vi "Actor Core.vi"(8 "error in":errorcluster, 11 "Supervisor in":refnum<class "Supervisor.lvclass">) -> (0 "error out":errorcluster, 3 "Actor out":refnum<class "Actor.lvclass">)   [LabVIEW 2020, in "Supervisor.lvlib" / "Supervisor.lvclass"]
doc: "<p>(<strong>Filename</strong>: <span class=\"dnl\">Actor Framework.lvlib:Actor.lvclass:Actor Core.vi</span>)</p>\n<p>Receives messages to the actor, reacts to them, and initiates any error handling that may shut the actor down.</p>\n<p>Descendant classes may override this VI to append parallel tasks for the actor to complete while it handles messages. Overrides use the <a href=\"nihelplauncher://docs/csh?context=lvcore_glang_udclass\">Call Parent Class Method</a> node.</p>"
uses:
  Supervisor.lvclass
  C:/Program Files/National Instruments/LabVIEW 2026/vi.lib/ActorFramework/Actor/Actor.lvclass
  <vilib>/ActorFramework/Actor/Actor.lvclass
  DAQ AI/DAQ AI/DAQ AI.lvclass
  DAQ DI/DAQ DI/DAQ DI.lvclass
  UI/UI/UI.lvclass
  <vilib>/ActorFramework/Message Enqueuer/Message Enqueuer.lvclass
  <vilib>/ActorFramework/Actor/Actor.lvclass/Actor.ctl
  <vilib>/ActorFramework/Message Enqueuer/Message Enqueuer.lvclass/Message Enqueuer.ctl
  Supervisor.lvclass/Supervisor.ctl
  DAQ AI/DAQ AI Messages/Threshold Msg/Threshold Msg.lvclass/Threshold Msg.ctl
  UI/UI Messages/Waveform Msg/Waveform Msg.lvclass/Waveform Msg.ctl
  UI/UI Messages/Status Msg/Status Msg.lvclass/Status Msg.ctl
  DAQ AI/DAQ AI Messages/Threshold Msg/Threshold Msg.lvclass
  C:/Program Files/National Instruments/LabVIEW 2026/vi.lib/ActorFramework/Message/Message.lvclass
  UI/UI Messages/Waveform Msg/Waveform Msg.lvclass
  UI/UI Messages/Status Msg/Status Msg.lvclass
  UI/UI Messages/Over Threshold Msg/Over Threshold Msg.lvclass
  DAQ DI/DAQ DI Messages/Acquire Status Msg/Acquire Status Msg.lvclass
  C:/Users/taacr/OneDrive/HP/Local/Actor Framework/Supervisor/Supervisor/Supervisor.lvclass
  C:/Users/taacr/OneDrive/HP/Local/Actor Framework/UI/UI/UI.lvclass
  C:/Users/taacr/OneDrive/HP/Local/Actor Framework/DAQ AI/DAQ AI/DAQ AI.lvclass
  C:/Users/taacr/OneDrive/HP/Local/Actor Framework/DAQ DI/DAQ DI/DAQ DI.lvclass
  TypeDef/Actor Queues.ctl
panel:
  out "Waveform Graph":waveform(dbl)[](graph)
  out "Threshold":dbl
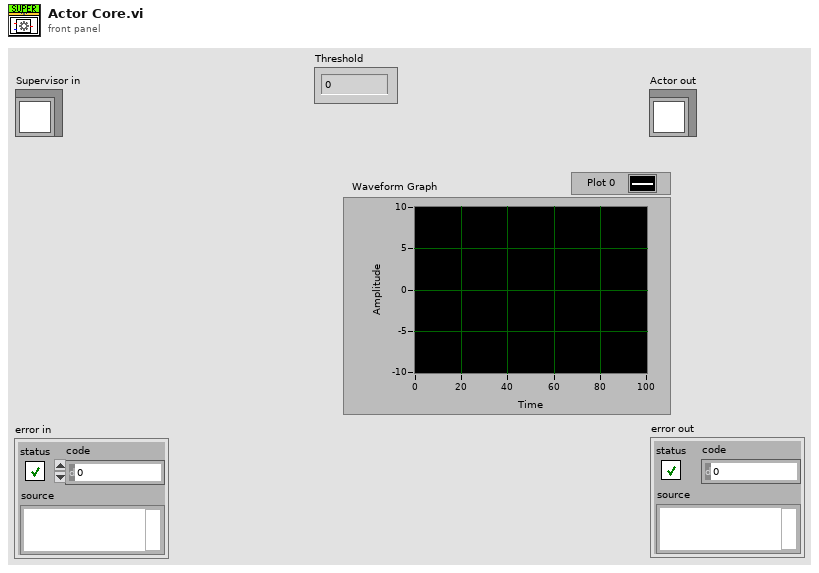
[diagram p1: front panel]
types:
  T1 = typedef "Supervisor.lvlib/Supervisor.lvclass/Actor Queues.ctl" = cluster{"Supervisor":refnum<class "Message Enqueuer.lvclass">, "UI":refnum<class "Message Enqueuer.lvclass">, "DAQ AI":refnum<class "Message Enqueuer.lvclass">, "DAQ DI":refnum<class "Message Enqueuer.lvclass">}
  T2 = typedef "Supervisor.lvlib/Supervisor.lvclass/User Events.ctl" = cluster{"Threshold Event":refnum<user-event>, "Waveform Graph Event":refnum<user-event>, "Status Event":refnum<user-event>, "Start/Stop Acquisition Event":refnum<user-event>, "Close UI Event":refnum<user-event>, "Stop Event":refnum<user-event>, "Over Threshold Event":refnum<user-event>}
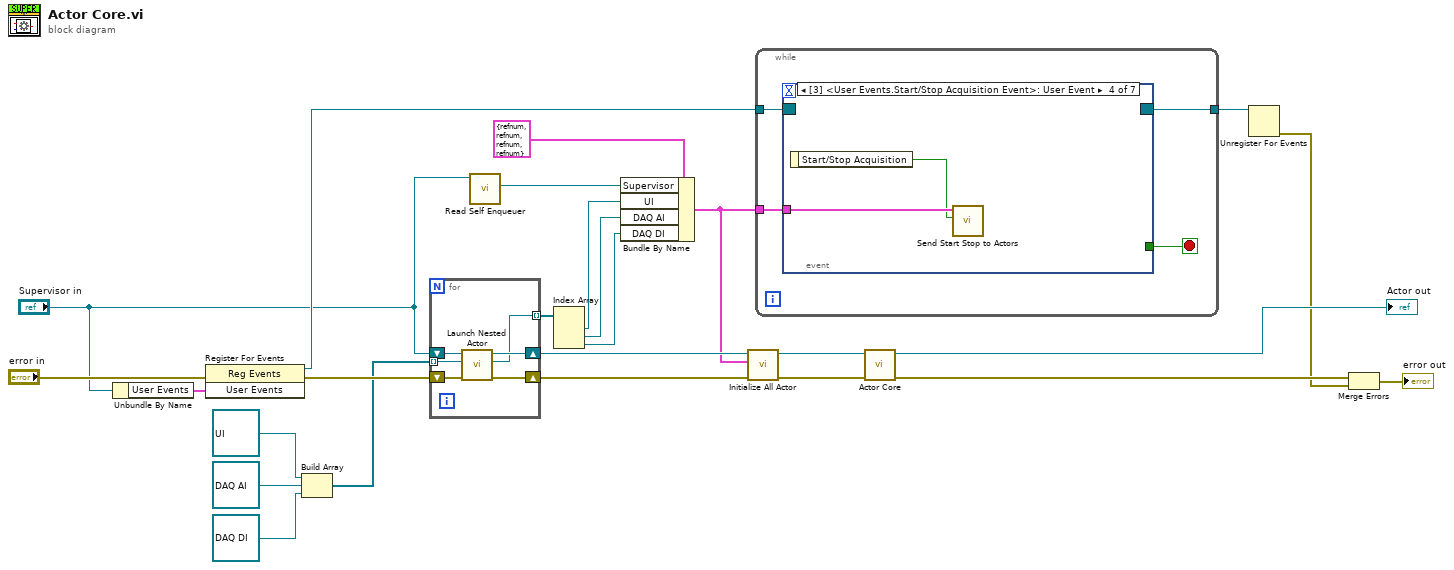
[diagram p0: block diagram]
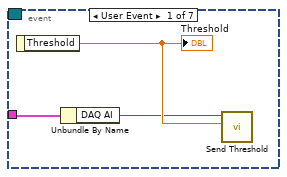
[diagram p2: hidden frame]
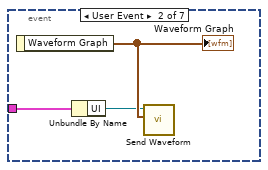
[diagram p3: hidden frame]
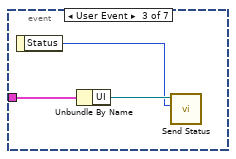
[diagram p4: hidden frame]
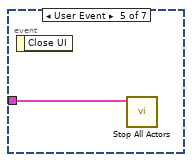
[diagram p5: hidden frame]
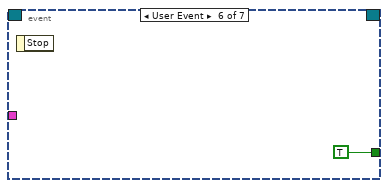
[diagram p6: hidden frame]
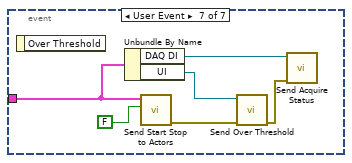
[diagram p7: hidden frame]
diagram:
  n1 = Unbundle By Name("Supervisor in") -> ("User Events"=w23:T2)
  n2 = register-events(error in="error in", w23) -> (reference out=w22:refnum<event-registration>, error out=w20:errorcluster)  [unwired: 1 in]
  n3 = Build Array(refnum<class "UI.lvclass"> refnum ("UI.lvlib:UI.lvclass"), refnum<class "DAQ AI.lvclass"> refnum ("DAQ AI.lvclass"), refnum<class "DAQ DI.lvclass"> refnum ("DAQ DI.lvlib:DAQ DI.lvclass")) -> (w19:refnum<class "Actor.lvclass">[])
  n4 = for {
    shift-right: [w29] -> w11
    shift-left: "Supervisor in" -> [w31]
    shift-right: [w28] -> w10
    shift-left: w20 -> [w30]
    tunnel: w19 -> [w27] mode=indexing
    tunnel: [w26] -> w15 mode=indexing
    n5 = call <vilib>:"Launch Nested Actor.vi"("error in (no error)"=w30, "Nested Actor"=w27, "Caller Actor in"=w31) -> ("error out"=w28:errorcluster, "Nested Actor's Enqueuer"=w26:refnum<class "Message Enqueuer.lvclass">, "Caller Actor out"=w29:refnum<class "Supervisor.lvclass">)  [unwired: 6 in]
  }
  n6 = call <vilib>:"Read Self Enqueuer.vi"("Actor"="Supervisor in") -> ("Self Enqueuer"=w16:refnum<class "Message Enqueuer.lvclass">)  [unwired: 10 in]
  n7 = Index Array(array=w15) -> (element #1=w14:refnum<class "Message Enqueuer.lvclass">, element #2=w13:refnum<class "Message Enqueuer.lvclass">, element #3=w12:refnum<class "Message Enqueuer.lvclass">)  [unwired: 3 in]
  n8 = Bundle By Name(cluster=T1 {"Supervisor"=refnum, "UI"=refnum, "DAQ AI"=refnum, "DAQ DI"=refnum} ("Actor Queue"), "Supervisor"=w16, "UI"=w14, "DAQ AI"=w13, "DAQ DI"=w12) -> (w7:T1)
  n9 = call "Initialize All Actor.vi"("error in (no error)"=w10, "Actor Queues"=w7, "Supervisor in"=w11) -> ("error out"=w8:errorcluster, "Supervisor out"=w9:refnum<class "Supervisor.lvclass">)  [unwired: 7 in]
  n10 = while {
    tunnel: w22 -> [w35]
    tunnel: w7 -> [w34]
    tunnel: [w33] -> w6
    stop <- w32 stop-if-true
    n11 = event shown="[3] <User Events.Start/Stop Acquisition Event>: User Event" {
      selector: w35 -> [_ _ _ _ _ _ _]
      dyn-events: [_ _ _ _ _ _ _] -> w33
      timeout: _ -> [_ _ _ _ _ _ _]
      tunnel: w34 -> [w37 w40 w44 w46 w47 _ w53]
      tunnel: [_ _ _ _ _ TRUE _] -> w32
      event User Event {
        n12 = event-data() -> ("Threshold"=w38:dbl)  [unwired: 1 in]
        "Threshold" <- w38
        n13 = Unbundle By Name(w37) -> ("DAQ AI"=w36:refnum<class "Message Enqueuer.lvclass">)
        n14 = call "Send Threshold.vi"("Threshold"=w38, "Message Enqueuer"=w36) -> ()  [unwired: 8 in, 2 out]
      }
      event User Event {
        n15 = event-data() -> ("Waveform Graph"=w41:waveform(dbl)[])  [unwired: 1 in]
        "Waveform Graph" <- w41
        n16 = Unbundle By Name(w40) -> ("UI"=w39:refnum<class "Message Enqueuer.lvclass">)
        n17 = call "Send Waveform.vi"("Waveform Graph"=w41, "Message Enqueuer"=w39) -> ()  [unwired: 8 in, 2 out]
      }
      event User Event {
        n18 = event-data() -> ("Status"=w42:u8)  [unwired: 1 in]
        n19 = Unbundle By Name(w44) -> ("UI"=w43:refnum<class "Message Enqueuer.lvclass">)
        n20 = call "Send Status.vi"("Status"=w42, "Message Enqueuer"=w43) -> ()  [unwired: 8 in, 2 out]
      }
      event User Event {
        n21 = event-data() -> ("Start/Stop Acquisition"=w45:bool)  [unwired: 1 in]
        n22 = call "Send Start Stop to Actors.vi"("Start/Stop Acquisition"=w45, "Actor Queues"=w46) -> ()  [unwired: 9 in, 1 out]
      }
      event User Event {
        n23 = event-data() -> ()  [unwired: 1 in, 1 out]
        n24 = call "Stop All Actors.vi"("input cluster"=w47) -> ()  [unwired: 10 in, 1 out]
      }
      event User Event {
        n25 = event-data() -> ()  [unwired: 1 in, 1 out]
      }
      event User Event {
        n26 = event-data() -> ()  [unwired: 1 in, 1 out]
        n27 = Unbundle By Name(w53) -> ("DAQ DI"=w50:refnum<class "Message Enqueuer.lvclass">, "UI"=w52:refnum<class "Message Enqueuer.lvclass">)
        n28 = call "Send Start Stop to Actors.vi"("Start/Stop Acquisition"=FALSE, "Actor Queues"=w53) -> ("error out"=w51:errorcluster)  [unwired: 9 in]
        n29 = call "Send Over Threshold.vi"("error in (no error)"=w51, "Message Enqueuer"=w52) -> ("error out"=w49:errorcluster)  [unwired: 8 in, 1 out]
        n30 = call "Send Acquire Status.vi"("error in (no error)"=w49, "Message Enqueuer"=w50) -> ()  [unwired: 8 in, 2 out]
      }
    }
  }
  n31 = call-parent "Actor Core.vi"("error in"=w8, "Actor in"=w9) -> ("error out"=w5:errorcluster, "Actor out"=→"Actor out":refnum<class "Actor.lvclass">)  [unwired: 8 in]
  n32 = Unregister For Events(event registration refnum=w6) -> (error out=w4:errorcluster)  [unwired: 1 in]
  n33 = Merge Errors(w5, w4) -> (→"error out":errorcluster)
